vi "Analyze MotorTest Datalog File.vi"() -> ()   [LabVIEW 2016]
uses:
  <vilib>/Utility/file.llb/Read Delimited Spreadsheet (DBL).vi
panel:
  out "XY Graph":cluster{"all rows":dbl[], "all rows":dbl[]}(graph)
  out "subarray 2":dbl[](array[numeric])
  out "subarray":dbl[](array[numeric])
  in  "delimiter (\\t)":string="\t"
  out "all rows":dbl[][](array[numeric])
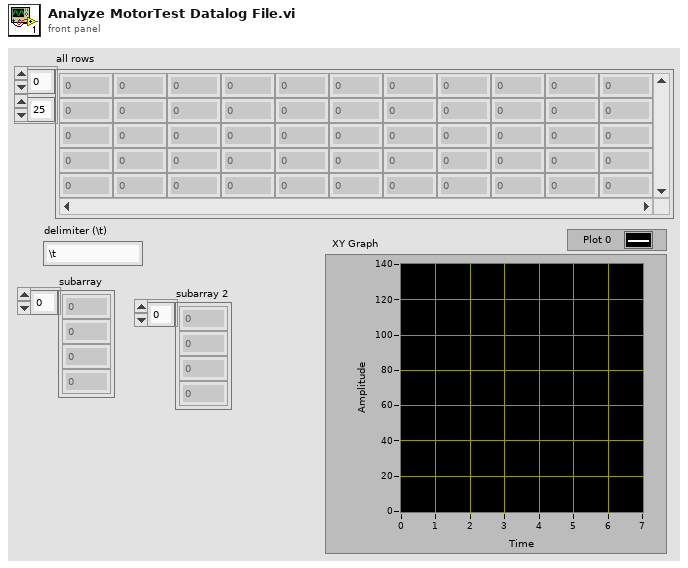
[diagram p1: front panel]
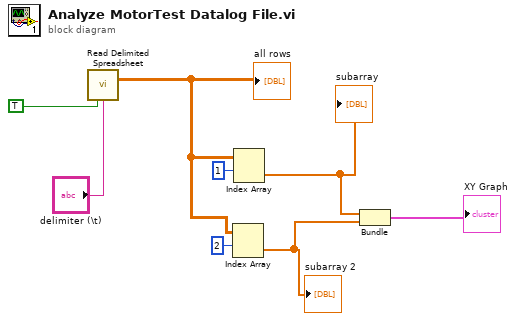
[diagram p0: block diagram]
diagram:
  n1 = call-poly <vilib>:"Read Delimited Spreadsheet.vi"("transpose? (F)"=TRUE, "delimiter (\\t)"="delimiter (\\t)") -> ("all rows"=w4:dbl[][])  [unwired: 8 in, 5 out]
  "all rows" <- w4
  n2 = Index Array(array=w4, index (row)=2) -> (element=w2:dbl[])  [unwired: 1 in]
  "subarray 2" <- w2
  n3 = Index Array(array=w4, index (row)=1) -> (element=w3:dbl[])  [unwired: 1 in]
  "subarray" <- w3
  n4 = Bundle("all rows"=w3, "all rows"=w2) -> (→"XY Graph":cluster{"all rows":dbl[], "all rows":dbl[]})  [unwired: 1 in]
